vi "Function_Result Table.vi"(7 "Result Action":T2, 9 "Result Array":T1(array[cluster]), 10 "Item Name":string, 11 "Result Table":refnum<vi>) -> ()   [LabVIEW 2013]
uses:
  Control/Control_Result Table Action #.ctl
  <vilib>/Utility/miscctls.llb/LVRowAndColumnTypeDef.ctl
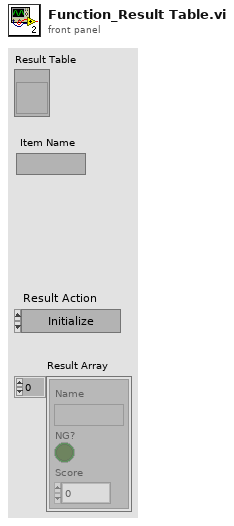
[diagram p1: front panel]
types:
  T1 = cluster{"Name":string, "NG?":bool, "Score":dbl}[]
  T2 = typedef "Control_Result Table Action #.ctl" = enum16{"Initialize", "Create Item", "Delete Item", "Set Result", "Idle"}
  T3 = typedef "LVRowAndColumnTypeDef.ctl" = cluster{"Row":i32, "Column":i32}
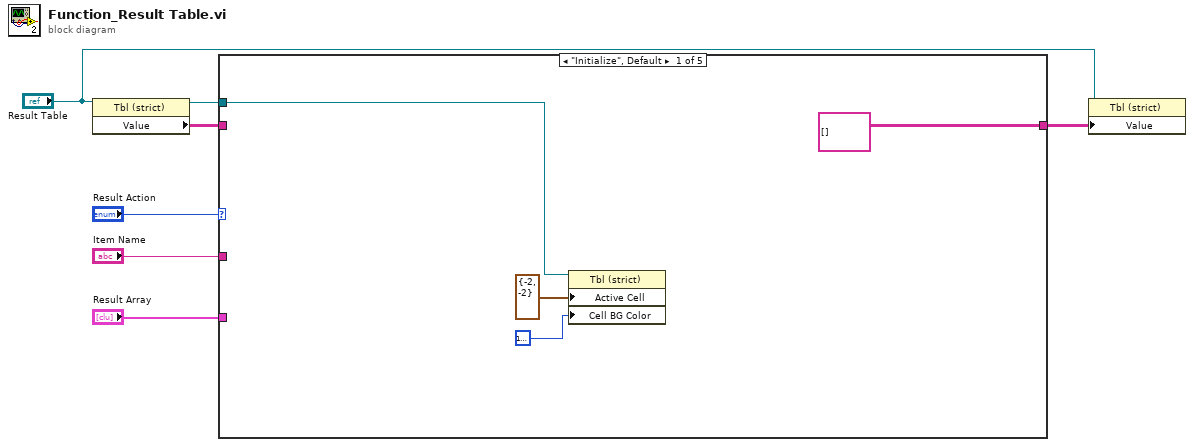
[diagram p0: block diagram]
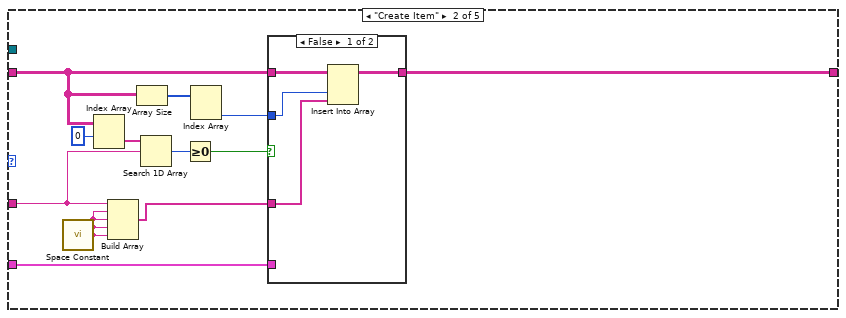
[diagram p2: hidden frame]
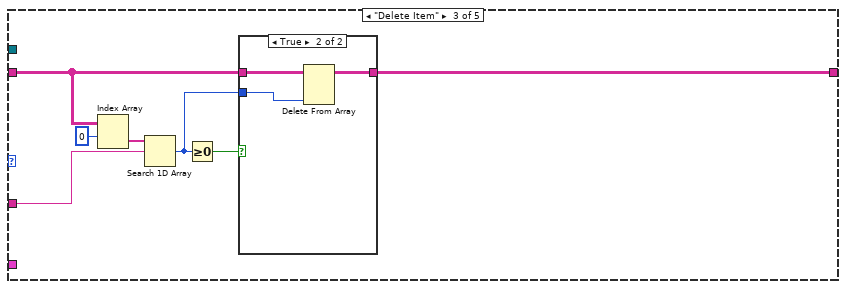
[diagram p4: hidden frame]
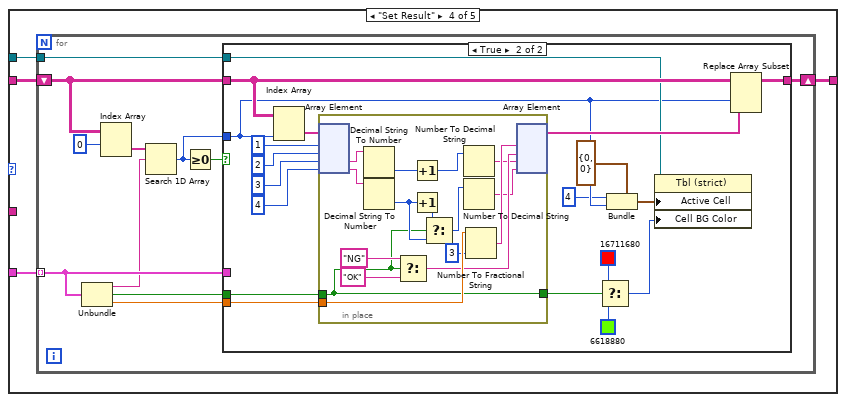
[diagram p6: hidden frame]
diagram:
  n1 = property class="Tbl (strict)"(reference="Result Table") -> (reference out=w1:refnum<vi>, "Value"=w4:string[][])  [unwired: 1 in, 1 out]
  n2 = case shown="\"Initialize\", Default" "Result Action" {
    tunnel: w4 -> [_ w16 w31 w42 w91]
    tunnel: [string[][] [] ("Value") w20 w29 w41 w91] -> w3
    tunnel: "Item Name" -> [_ w18 w30 _ _]
    tunnel: "Result Array" -> [_ w19 _ w43 _]
    tunnel: w1 -> [w8 _ _ w40 _]
    frame "Initialize", Default {
      n3 = property class="Tbl (strict)"(reference=w8, "Active Cell"=T3 {"Row"=-2, "Column"=-2} ("Active Cell:Active Cell"), "Cell BG Color"=u32 16777225 ("Color Box")) -> ()  [unwired: 1 in, 2 out]
    }
    frame "Create Item" {
      n4 = call <vilib>:"Space Constant.vi"() -> ("String"=w12:string)
      n5 = Index Array(array=w16, index (row)=0) -> (element=w22:string[])  [unwired: 1 in]
      n6 = Build Array(w18, w12, w12, w12, w12) -> (w17:string[])
      n7 = Array Size(array=w16) -> (size(s)=w15:i32[])
      n8 = Search 1D Array(1D array=w22, element=w18) -> (index of element=w13:i32)  [unwired: 1 in]
      n9 = Greater Or Equal To 0?(x=w13) -> (x >= 0?=w21:bool)
      n10 = Index Array(array=w15) -> (element #2=w14:i32)  [unwired: 2 in, 1 out]
      n11 = case shown="False" w21 {
        tunnel: w16 -> [w27 w28]
        tunnel: [w26 w28] -> w20
        tunnel: w17 -> [w25 _]
        tunnel: w19 -> [_ _]
        tunnel: w14 -> [w24 _]
        frame False {
          n12 = Insert Into Array(array=w27, index (col)=w24, new element=w25) -> (w26:string[][])  [unwired: 1 in]
        }
        frame True {
        }
      }
    }
    frame "Delete Item" {
      n13 = Index Array(array=w31, index (row)=0) -> (element=w34:string[])  [unwired: 1 in]
      n14 = Search 1D Array(1D array=w34, element=w30) -> (index of element=w32:i32)  [unwired: 1 in]
      n15 = Greater Or Equal To 0?(x=w32) -> (x >= 0?=w33:bool)
      n16 = case shown="True" w33 {
        tunnel: w31 -> [w36 w39]
        tunnel: [w36 w38] -> w29
        tunnel: w32 -> [_ w37]
        frame False {
        }
        frame True {
          n17 = Delete From Array(array=w39, index (col)=w37) -> (array with subset deleted=w38:string[][])  [unwired: 2 in, 1 out]
        }
      }
    }
    frame "Set Result" {
      n18 = for {
        tunnel: w43 -> [w48] mode=indexing
        shift-right: [w49] -> w41
        shift-left: w42 -> [w50]
        tunnel: w40 -> [w44]
        n19 = Unbundle(w48) -> ("Name"=w45:string, "NG?"=w46:bool, "Score"=w47:dbl)
        n20 = Index Array(array=w50, index (row)=0) -> (element=w53:string[])  [unwired: 1 in]
        n21 = Search 1D Array(1D array=w53, element=w45) -> (index of element=w51:i32)  [unwired: 1 in]
        n22 = Greater Or Equal To 0?(x=w51) -> (x >= 0?=w52:bool)
        n23 = case shown="True" w52 {
          tunnel: w50 -> [w55 w66]
          tunnel: [w55 w67] -> w49
          tunnel: w51 -> [_ w63]
          tunnel: w48 -> [_ _]
          tunnel: w47 -> [_ w69]
          tunnel: w46 -> [_ w70]
          tunnel: w44 -> [_ w64]
          frame False {
          }
          frame True {
            n24 = Index Array(array=w66, index (col)=w63) -> (element=w74:string[])  [unwired: 1 in]
            n25 = in-place {
              in-place-border: w70 -> [w75]
              in-place-border: w69 -> [w90]
              in-place-border: [w75] -> w57
              n26 = in-place-array #1(w74, 1, 2, 3, 4) -> (w84:string, w83:string)  [unwired: 2 out]
              n27 = Decimal String To Number(string=w84) -> (number=w82:i32)  [unwired: 2 in, 1 out]
              n28 = Decimal String To Number(string=w83) -> (number=w76:i32)  [unwired: 2 in, 1 out]
              n29 = Select(t="NG", s=w75, f="OK") -> (s? t:f=w87:string)
              n30 = Increment(x=w82) -> (x+1=w81:i32)
              n31 = Increment(x=w76) -> (x+1=w77:i32)
              n32 = Select(t=w77, s=w75, f=w76) -> (s? t:f=w78:i32)
              n33 = Number To Decimal String(number=w81) -> (decimal integer string=w80:string)  [unwired: 1 in]
              n34 = Number To Decimal String(number=w78) -> (decimal integer string=w79:string)  [unwired: 1 in]
              n35 = Number To Fractional String(number=w90, precision (6)=i16 3) -> (F-format string=w89:string)  [unwired: 2 in]
              n36 = in-place-array #1(w89, w87, w80, w79) -> (w65:string[])  [unwired: 4 out]
            }
            n37 = Select(t=u32 16711680 ("Color Box"), s=w57, f=u32 6618880 ("Color Box")) -> (s? t:f=w59:u32)
            n38 = Bundle(cluster=T3 {"Row"=0, "Column"=0} ("Active Cell:Active Cell"), "Row"=4, "Column"=w63) -> (w60:T3)
            n39 = property class="Tbl (strict)"(reference=w64, "Active Cell"=w60, "Cell BG Color"=w59) -> ()  [unwired: 1 in, 2 out]
            n40 = Replace Array Subset(array=w66, new element=w65, index (col)=w63) -> (w67:string[][])  [unwired: 1 in]
          }
        }
      }
    }
    frame "Idle" {
    }
  }
  n41 = property class="Tbl (strict)"(reference="Result Table", "Value"=w3) -> ()  [unwired: 1 in, 2 out]
